vi "Begin.vi"(8 "error in":errorcluster) -> (0 "error out":errorcluster)   [LabVIEW 2018]
doc: "Called before other user functions, this VI is expected to open initial I/O refnums, load in file data, and do all program initialization. Notice that the <B>error out</B> terminal is simply used for data flow. Wiring it to other structures or subVIs ensures that this VI runs first."
uses:
  <vilib>/Rock Robotics/WPI/Joystick/WPI_JoystickDeviceEnum.ctl
  Joystick.ctl
  LeftMotors.ctl
  RightMotors.ctl
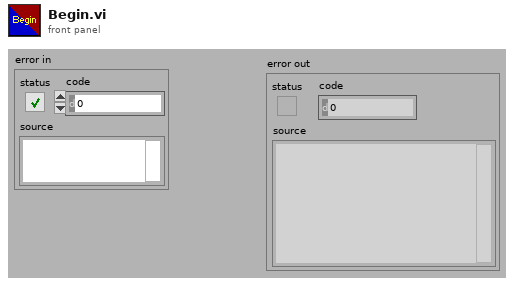
[diagram p1: front panel]
types:
  T1 = typedef "RightMotors.ctl" = enum16{"Right Motor 1", "Right Motor 2", "Right Motor 3"}
  T2 = typedef "LeftMotors.ctl" = enum16{"LeftMotor1", "LeftMotor2", "LeftMotor3"}
  T3 = typedef "Joystick.ctl" = enum16{"Joystick"}
  T4 = typedef "WPI_JoystickDeviceEnum.ctl" = enum16{"USB 0", "USB 1", "USB 2", "USB 3", "USB 4", "USB 5"}
  T5 = typedef "WPI_JoystickDevRef.ctl" = cluster{"Device":T4}
  T6 = typedef "WPI_MotorControlDeviceRef.ctl" = cluster{"DeviceStatus":errorcluster, "Type":T7, "PWM":cluster{"PWM Channel":T8, "DeadBand":T9}, "CAN":cluster{"Device Number":u8, "SetOutput VI Ref":variant, "GetOutput VI Ref":variant, "Enable VI Ref":variant, "Disable VI Ref":variant, "Data":variant}, "Invert":bool, "DIO PWM":cluster{"PWM \"Enable\" Channel":T8, "DIOChannel":T10, "PWM Rate":dbl}}
  T7 = typedef "WPI_MotorControlType.ctl" = enum16{"PWM", "CAN", "DIO PWM"}
  T8 = typedef "FPGA_DIOPWMChannel.ctl" = enum8{"PWM 0", "PWM 1", "PWM 2", "PWM 3", "PWM 4", "PWM 5", "PWM 6", "PWM 7", "PWM 8", "PWM 9", "PWM MXP 0", "PWM MXP 1", "PWM MXP 2", "PWM MXP 3", "PWM MXP 4", "PWM MXP 5", "PWM MXP 6", "PWM MXP 7", "PWM MXP 8", "PWM MXP 9", "Invalid"}
  T9 = typedef "WPI_PWMDeadband.ctl" = cluster{"Name":string, "maxPositivePwm":i32, "minPositivePwm":i32, "centerPwm":i32, "maxNegativePwm":i32, "minNegativePwm":i32, "angularRange":u16}
  T10 = typedef "FPGA_DIOChannel.ctl" = enum8{"DIO 0", "DIO 1", "DIO 2", "DIO 3", "DIO 4", "DIO 5", "DIO 6", "DIO 7", "DIO 8", "DIO 9", "DIO MXP 0", "DIO MXP 1", "DIO MXP 2", "DIO MXP 3", "DIO MXP 4", "DIO MXP 5", "DIO MXP 6", "DIO MXP 7", "DIO MXP 8", "DIO MXP 9", "DIO MXP 10", "DIO MXP 11", "DIO MXP 12", "DIO MXP 13", "DIO MXP 14", "DIO MXP 15", "SPI Port CS1", "SPI Port CS2", "SPI Port CS3", "SPI Port MISO", "SPI Port MOSI", "Invalid"}
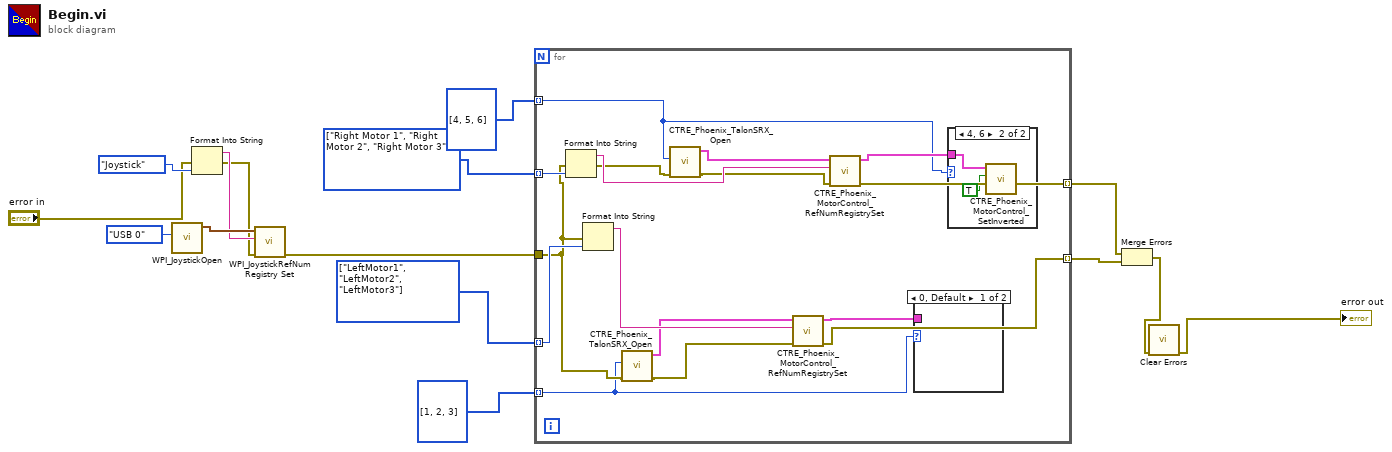
[diagram p0: block diagram]
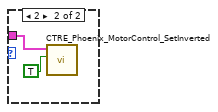
[diagram p2: hidden frame]
diagram:
  w7 = T1[] [enum."Right Motor 1", enum."Right Motor 2", enum."Right Motor 3"] items=["Right Motor 1", "Right Motor 2", "Right Motor 3"] ("Array")
  w8 = T2[] [enum."LeftMotor1", enum."LeftMotor2", enum."LeftMotor3"] items=["LeftMotor1", "LeftMotor2", "LeftMotor3"] ("Array")
  n1 = call <vilib>:"WPI_JoystickOpen.vi"("JoystickDevice"=WPI_JoystickDeviceEnum."USB 0") -> ("JoystickDevRef"=w14:T5)  [unwired: 10 in]
  n2 = Format Into String(error in="error in", Joystick."Joystick") -> (resulting string=w12:string, error out=w11:errorcluster)  [unwired: 2 in]
  n3 = call <vilib>:"WPI_JoystickRefNum Registry Set.vi"("error in (no error)"=w11, "refnum name"=w12, "JoystickDevRef"=w14) -> ("error out"=w10:errorcluster)  [unwired: 7 in, 1 out]
  n4 = for {
    tunnel: w8 -> [w31] mode=indexing
    tunnel: w10 -> [w23]
    tunnel: [w26] -> w9 mode=indexing
    tunnel: w7 -> [w29] mode=indexing
    tunnel: [w27] -> w6 mode=indexing
    tunnel: u8[] [1, 2, 3] ("Device Number") -> [w16] mode=indexing
    tunnel: u8[] [4, 5, 6] ("Device Number") -> [w18] mode=indexing
    n5 = Format Into String(error in=w23, w29) -> (resulting string=w28:string, error out=w20:errorcluster)  [unwired: 2 in]
    n6 = Format Into String(error in=w23, w31) -> (resulting string=w30:string)  [unwired: 2 in, 1 out]
    n7 = call <vilib>:"CTRE_Phoenix_TalonSRX_Open.vi"("error in"=w23, "Device Number"=w16) -> ("error out"=w24:errorcluster, "CAN Talon SRX Ref"=w25:T6)  [unwired: 8 in]
    n8 = call <vilib>:"CTRE_Phoenix_TalonSRX_Open.vi"("error in"=w20, "Device Number"=w18) -> ("error out"=w21:errorcluster, "CAN Talon SRX Ref"=w22:T6)  [unwired: 8 in]
    n9 = call <vilib>:"CTRE_Phoenix_MotorControl_RefNumRegistrySet.vi"("error in (no error)"=w24, "refnum name"=w30, "PhoenixMotorControlDevRef"=w25) -> ("error out"=w26:errorcluster, "PhoenixMotorControlDevRef"=w17:T6)  [unwired: 7 in]
    n10 = call <vilib>:"CTRE_Phoenix_MotorControl_RefNumRegistrySet.vi"("error in (no error)"=w21, "refnum name"=w28, "PhoenixMotorControlDevRef"=w22) -> ("error out"=w27:errorcluster, "PhoenixMotorControlDevRef"=w19:T6)  [unwired: 7 in]
    n11 = case shown="0, Default" w16 {
      tunnel: w17 -> [_ w33]
      frame 0, Default {
      }
      frame 2 {
        n12 = call <vilib>:"CTRE_Phoenix_MotorControl_SetInverted.vi"("Invert?"=TRUE, "PhoenixMotorControlDevRef"=w33) -> ()  [unwired: 8 in, 2 out]
      }
    }
    n13 = case shown="4, 6" w18 {
      tunnel: w19 -> [_ w35]
      frame 0, Default {
      }
      frame 4, 6 {
        n14 = call <vilib>:"CTRE_Phoenix_MotorControl_SetInverted.vi"("Invert?"=TRUE, "PhoenixMotorControlDevRef"=w35) -> ()  [unwired: 8 in, 2 out]
      }
    }
  }
  n15 = Merge Errors(w6, w9) -> (w3:errorcluster)
  n16 = call <vilib>:"Clear Errors.vi"("error in (no error)"=w3) -> ("error out"=→"error out":errorcluster)  [unwired: 5 in, 1 out]
